vi "oax_Condition Tach Signal.vi"(11 "tach in":dbl[](array[numeric])) -> (3 "tach out":dbl[](array[numeric]))   [LabVIEW 2017]
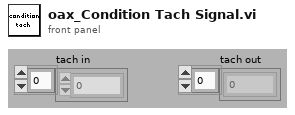
[diagram p1: front panel]
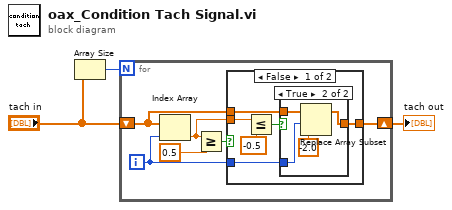
[diagram p0: block diagram]
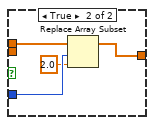
[diagram p3: hidden frame]
diagram:
  n1 = Array Size(array="tach in") -> (size(s)=w1:i32)
  n2 = for {
    N: w1 -> [_]
    shift-right: [w5] -> w3
    shift-left: "tach in" -> [w7]
    i -> [w6]
    n3 = Index Array(array=w7, index=w6) -> (element=w4:dbl)
    n4 = Greater Or Equal?(x=w4, y=0.5) -> (x >= y?=w8:bool)
    n5 = case shown="False" w8 {
      tunnel: w7 -> [w11 w24]
      tunnel: w6 -> [w10 w23]
      tunnel: [w12 w21] -> w5
      tunnel: w4 -> [w14 _]
      frame False {
        n6 = Less Or Equal?(x=w14, y=-0.5) -> (x <= y?=w13:bool)
        n7 = case shown="True" w13 {
          tunnel: [w16 w19] -> w12
          tunnel: w11 -> [w16 w20]
          tunnel: w10 -> [_ w18]
          frame False {
          }
          frame True {
            n8 = Replace Array Subset(array=w20, new element=-2.0 ("y"), index=w18) -> (w19:dbl[])
          }
        }
      }
      frame True {
        n9 = Replace Array Subset(array=w24, new element=2.0 ("new element/subarray"), index=w23) -> (w21:dbl[])
      }
    }
  }
  "tach out" <- w3
